vi "Autonomous Independent.vi"() -> ()   [LabVIEW 2014]
doc: "This VI is called when autonomous begins, and will automatically be terminated when autonomous ends. You can carry out timed or sensor driven robot movement independently without needing to return to the caller."
uses:
  <vilib>/Rock Robotics/WPI/Joystick/WPI_JoystickGetSetRefNum.vi
  <vilib>/Rock Robotics/Network Tables/SD Write Numeric Array.vi
  <vilib>/Rock Robotics/Network Tables/SD Read Number.vi
  <vilib>/Rock Robotics/WPI/RobotDrive/WPI_RobotDriveGetSetRefNum.vi
  <vilib>/Rock Robotics/WPI/RobotDrive/WPI_RobotDriveMecanumDrive_Cartesian.vi
panel:
  out "Current Movement, for debugging":T1 {"Z Joystick Value" scale=-1.0..1.0; "Y Joystick Value" scale=1.0..-1.0; "X Joystick Value" scale=-1.0..1.0}
  in  "Array of robot movements":T2(array[cluster]) {"Z Joystick Value" scale=-1.0..1.0; "Y Joystick Value" scale=1.0..-1.0; "X Joystick Value" scale=-1.0..1.0}
  # "Be sure to right-click and choose Data Operations>>Make Current Value default if you want to save the array values with the VI"
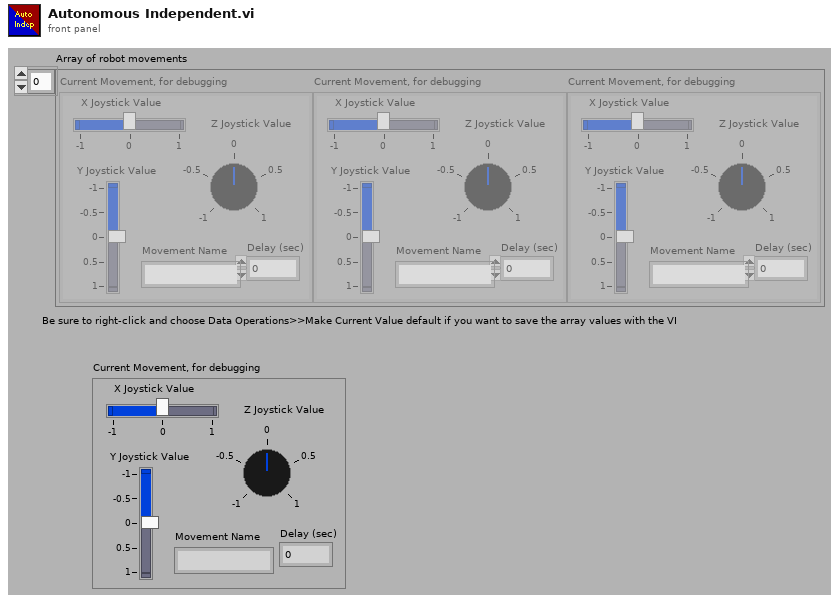
[diagram p1: front panel]
types:
  T1 = cluster{"X Joystick Value":dbl, "Y Joystick Value":dbl, "Z Joystick Value":dbl, "Delay (sec)":dbl, "Movement Name":string}
  T2 = cluster{"X Joystick Value":dbl, "Y Joystick Value":dbl, "Z Joystick Value":dbl, "Delay (sec)":dbl, "Movement Name":string}[]
  T3 = typedef "WPI_JoystickDevRef.ctl" = cluster{"Device":T4}
  T4 = typedef "WPI_JoystickDeviceEnum.ctl" = enum16{"USB 0", "USB 1", "USB 2", "USB 3", "USB 4", "USB 5"}
  T5 = typedef "WPI_RobotDriveDevRef.ctl" = cluster{"DevStatus":errorcluster, "Motors[]":T6[], "Square Inputs":bool, "Max Output":dbl}
  T6 = typedef "WPI_MotorControlDeviceRef.ctl" = cluster{"DeviceStatus":errorcluster, "Type":T7, "PWM":cluster{"Controller":T8, "PWM Channel":T9, "DeadBand":T10}, "CAN":cluster{"Device Number":u8, "Control Mode":T11, "Semaphore":T12, "Max Vout":dbl, "TalonSRX Control Mode":T13}, "Invert":bool, "TransformRef":T14, "InvTransformRef":T14}
  T7 = typedef "WPI_MotorControlType.ctl" = enum16{"PWM", "CAN", "CANTalonSRX"}
  T8 = typedef "FPGA_TypedefDigitalModule.ctl" = enum16{"Controller 1"}
  T9 = typedef "FPGA_DIOPWMChannel.ctl" = enum8{"PWM 0", "PWM 1", "PWM 2", "PWM 3", "PWM 4", "PWM 5", "PWM 6", "PWM 7", "PWM 8", "PWM 9", "PWM MXP 0", "PWM MXP 1", "PWM MXP 2", "PWM MXP 3", "PWM MXP 4", "PWM MXP 5", "PWM MXP 6", "PWM MXP 7", "PWM MXP 8", "PWM MXP 9", "Invalid"}
  T10 = typedef "WPI_PWMDeadband.ctl" = cluster{"Name":string, "maxPositivePwm":i32, "minPositivePwm":i32, "centerPwm":i32, "maxNegativePwm":i32, "minNegativePwm":i32, "angularRange":u16}
  T11 = typedef "WPI_CANJaguar_ControlMode.ctl" = enum8{"Percent VBus", "Current", "Speed", "Position", "Voltage"}
  T12 = typedef "Semaphore RefNum" = refnum<k1>
  T13 = typedef "WPI_CANTalonSRX_APIControlMode.ctl" = enum8{"Percent VBus", "Speed", "Position", "Slave", "Unchanged / Invalid"}
  T14 = typedef "WPI_PWMTransform_ConPane.ctl" = refnum<vi>
  T15 = typedef "WPI_EncoderDevRef.ctl" = cluster{"DevStatus":errorcluster, "EncoderIndex":T16, "CounterIndex":T17, "DistancePerCount":dbl, "Decoding Type":T18}
  T16 = typedef "FPGA_EncoderIdx.ctl" = enum8{"Enc 0", "Enc 1", "Enc 2", "Enc 3", "Enc 4", "Enc 5", "Enc 6", "Enc 7", "Invalid"}
  T17 = typedef "FPGA_CounterCtrSystemIndex.ctl" = enum8{"Ctr 0", "Ctr 1", "Ctr 2", "Ctr 3", "Ctr 4", "Ctr 5", "Ctr 6", "Ctr 7", "Invalid"}
  T18 = typedef "WPI_EncoderType.ctl" = enum16{"1x", "2x", "4x"}
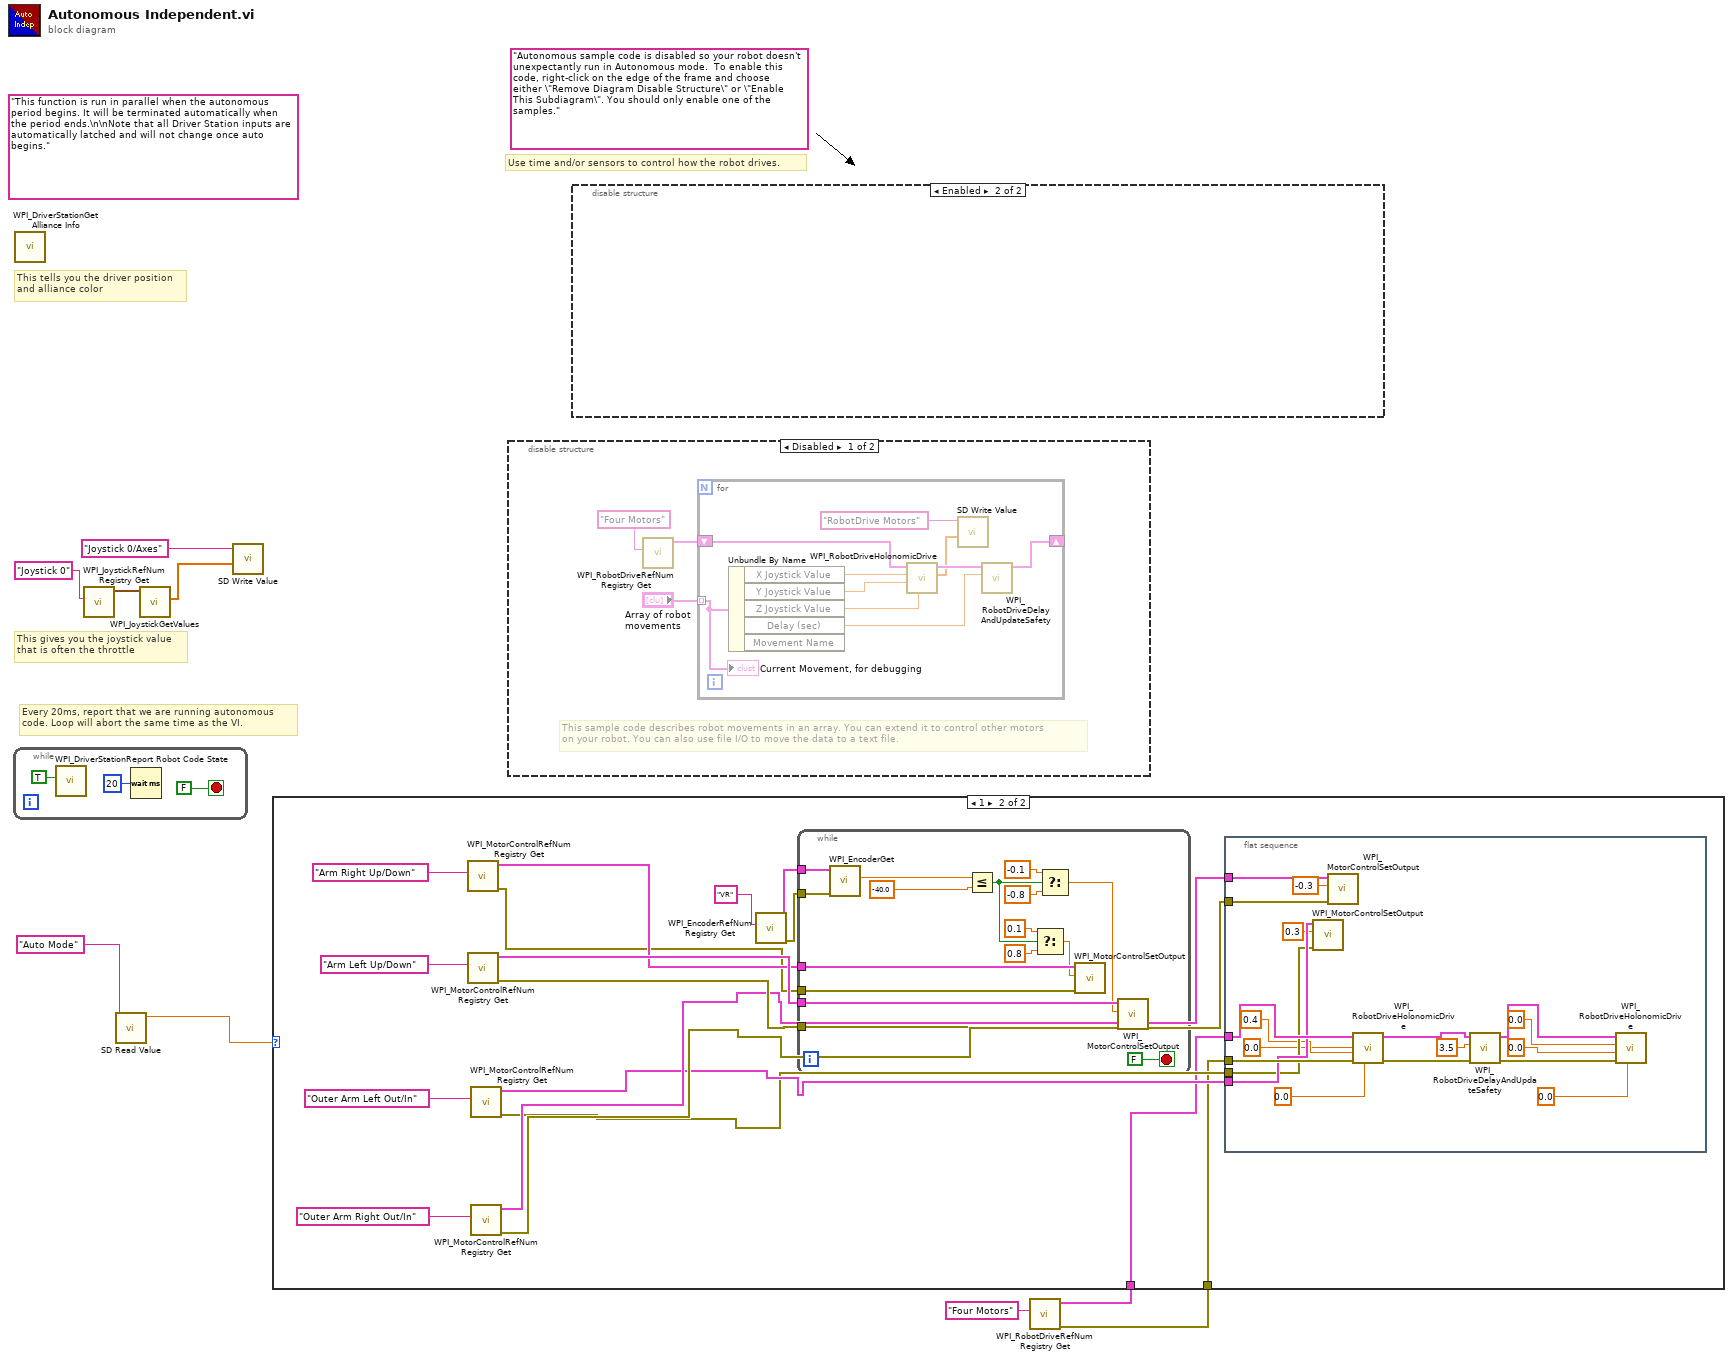
[diagram p0: block diagram]
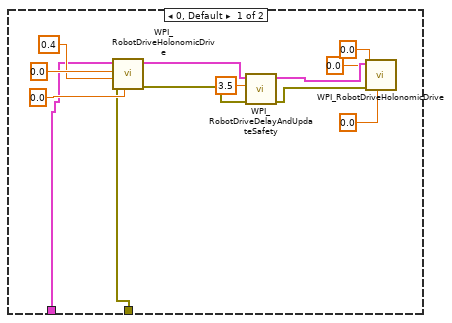
[diagram p2: hidden frame]
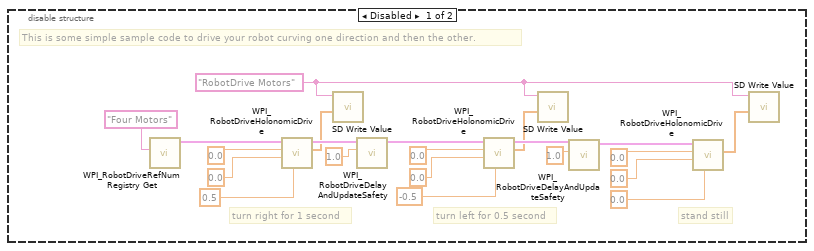
[diagram p4: hidden frame]
diagram:
  (unwired) "Autonomous sample code is disabled so your robot doesn't unexpectantly run in Autonomous mode.  To enable this code, right-click on the edge of the frame and choose either \"Remove Diagram Disable Structure\" or \"Enable This Subdiagram\". You should only enable one of the samples."
  (unwired) "This function is run in parallel when the autonomous period begins. It will be terminated automatically when the period ends.\n\nNote that all Driver Station inputs are automatically latched and will not change once auto begins."
  # "Every 20ms, report that we are running autonomous\ncode. Loop will abort the same time as the VI."
  # "This gives you the joystick value\nthat is often the throttle"
  # "Use time and/or sensors to control how the robot drives."
  # "This tells you the driver position\nand alliance color"
  n1 = while {
    stop <- FALSE stop-if-true
    n2 = call <vilib>:"WPI_DriverStationReport Robot Code State.vi"("Autonomous"=TRUE) -> ()  [unwired: 10 in, 1 out]
    n3 = Wait (ms)(milliseconds to wait=u32 20) -> ()  [unwired: 1 out]
  }
  n4 = call <vilib>:"WPI_DriverStationGet Alliance Info.vi"() -> ()  [unwired: 12 out]
  n5 = call <vilib>:"WPI_JoystickRefNum Registry Get.vi"("refnum name"="Joystick 0") -> ("JoystickDevRef"=w8:T3)  [unwired: 1 in, 9 out]
  n6 = call-poly <vilib>:"SD Read Value.vi"("Name"="Auto Mode") -> ("Numeric"=w5:dbl)  [unwired: 8 in, 2 out]
  n7 = call <vilib>:"WPI_JoystickGetValues.vi"("JoystickDevRef"=w8) -> ("Axes"=w6:dbl[])  [unwired: 6 in, 4 out]
  n8 = call-poly <vilib>:"SD Write Value.vi"("Numeric Array"=w6, "Name"="Joystick 0/Axes") -> ()  [unwired: 8 in, 2 out]
  n9 = disable-structure shown="Disabled" {
    frame Disabled {
      # "This sample code describes robot movements in an array. You can extend it to control other motors\non your robot. You can also use file I/O to move the data to a text file."
      n10 = call <vilib>:"WPI_RobotDriveRefNum Registry Get.vi"("refnum name"="Four Motors") -> ("RobotDriveDevRef"=w14:T5)  [unwired: 1 in, 9 out]
      n11 = for {
        shift-right: [w22] -> _
        shift-left: w14 -> [w23]
        tunnel: "Array of robot movements" -> [w18] mode=indexing
        n12 = Unbundle By Name(w18) -> ("X Joystick Value"=w21:dbl, "Y Joystick Value"=w20:dbl, "Z Joystick Value"=w17:dbl, "Delay (sec)"=w19:dbl)  [unwired: 1 out]
        n13 = call-poly <vilib>:"WPI_RobotDriveHolonomicDrive.vi"("Rotation"=w17, "Y"=w20, "X"=w21, "RobotDriveDevRef"=w23) -> ("Motor Values"=w16:dbl[], "RobotDriveDevRef"=w24:T5)  [unwired: 5 in, 1 out]
        n14 = call-poly <vilib>:"SD Write Value.vi"("Numeric Array"=w16, "Name"="RobotDrive Motors") -> ()  [unwired: 8 in, 2 out]
        n15 = call <vilib>:"WPI_RobotDriveDelayAndUpdateSafety.vi"("Delay (s)"=w19, "RobotDriveDevRef"=w24) -> ("RobotDriveDevRef 2"=w22:T5)  [unwired: 8 in, 1 out]
        "Current Movement, for debugging" <- w18
      }
    }
    frame Enabled {
    }
  }
  n16 = disable-structure shown="Enabled" {
    frame Disabled {
      w32 = "RobotDrive Motors" ("Name")
      # "This is some simple sample code to drive your robot curving one direction and then the other."
      # "stand still"
      # "turn left for 0.5 second"
      # "turn right for 1 second"
      n17 = call <vilib>:"WPI_RobotDriveRefNum Registry Get.vi"("refnum name"="Four Motors") -> ("RobotDriveDevRef"=w33:T5)  [unwired: 1 in, 9 out]
      n18 = call-poly <vilib>:"WPI_RobotDriveHolonomicDrive.vi"("Rotation"=0.5, "Y"=0.0 ("X axis value"), "X"=0.0 ("X axis value"), "RobotDriveDevRef"=w33) -> ("Motor Values"=w28:dbl[], "RobotDriveDevRef"=w40:T5)  [unwired: 5 in, 1 out]
      n19 = call-poly <vilib>:"SD Write Value.vi"("Numeric Array"=w28, "Name"=w32) -> ()  [unwired: 8 in, 2 out]
      n20 = call <vilib>:"WPI_RobotDriveDelayAndUpdateSafety.vi"("Delay (s)"=1.0, "RobotDriveDevRef"=w40) -> ("RobotDriveDevRef 2"=w39:T5)  [unwired: 8 in, 1 out]
      n21 = call-poly <vilib>:"WPI_RobotDriveHolonomicDrive.vi"("Rotation"=-0.5, "Y"=0.0 ("X axis value"), "X"=0.0 ("X axis value"), "RobotDriveDevRef"=w39) -> ("Motor Values"=w27:dbl[], "RobotDriveDevRef"=w38:T5)  [unwired: 5 in, 1 out]
      n22 = call-poly <vilib>:"SD Write Value.vi"("Numeric Array"=w27, "Name"=w32) -> ()  [unwired: 8 in, 2 out]
      n23 = call <vilib>:"WPI_RobotDriveDelayAndUpdateSafety.vi"("Delay (s)"=1.0, "RobotDriveDevRef"=w38) -> ("RobotDriveDevRef 2"=w37:T5)  [unwired: 8 in, 1 out]
      n24 = call-poly <vilib>:"WPI_RobotDriveHolonomicDrive.vi"("Rotation"=0.0 ("X axis value"), "Y"=0.0 ("X axis value"), "X"=0.0 ("X axis value"), "RobotDriveDevRef"=w37) -> ("Motor Values"=w26:dbl[])  [unwired: 5 in, 2 out]
      n25 = call-poly <vilib>:"SD Write Value.vi"("Numeric Array"=w26, "Name"=w32) -> ()  [unwired: 8 in, 2 out]
    }
    frame Enabled {
    }
  }
  n26 = call <vilib>:"WPI_RobotDriveRefNum Registry Get.vi"("refnum name"="Four Motors") -> ("error out"=w2:errorcluster, "RobotDriveDevRef"=w3:T5)  [unwired: 1 in, 8 out]
  n27 = case shown="1" w5 {
    tunnel: w3 -> [w48 w61]
    tunnel: w2 -> [w47 w60]
    frame 0, Default {
      n28 = call-poly <vilib>:"WPI_RobotDriveHolonomicDrive.vi"("Rotation"=0.0, "error in (no error)"=w47, "Y"=0.4 ("Magnitude"), "X"=0.0 ("Direction"), "RobotDriveDevRef"=w48) -> ("error out"=w57:errorcluster, "RobotDriveDevRef"=w56:T5)  [unwired: 4 in, 1 out]
      n29 = call <vilib>:"WPI_RobotDriveDelayAndUpdateSafety.vi"("error in (no error)"=w57, "Delay (s)"=3.5, "RobotDriveDevRef"=w56) -> ("error out"=w59:errorcluster, "RobotDriveDevRef 2"=w58:T5)  [unwired: 7 in]
      n30 = call-poly <vilib>:"WPI_RobotDriveHolonomicDrive.vi"("Rotation"=0.0, "error in (no error)"=w59, "Y"=0.0, "X"=0.0, "RobotDriveDevRef"=w58) -> ()  [unwired: 4 in, 3 out]
    }
    frame 1 {
      n31 = call <vilib>:"WPI_MotorControlRefNum Registry Get.vi"("refnum name"="Arm Right Up/Down") -> ("error out"=w69:errorcluster, "MotorControlDevRef"=w70:T6)  [unwired: 9 in]
      n32 = call <vilib>:"WPI_MotorControlRefNum Registry Get.vi"("refnum name"="Arm Left Up/Down") -> ("error out"=w72:errorcluster, "MotorControlDevRef"=w71:T6)  [unwired: 9 in]
      n33 = call <vilib>:"WPI_MotorControlRefNum Registry Get.vi"("refnum name"="Outer Arm Left Out/In") -> ("error out"=w62:errorcluster, "MotorControlDevRef"=w63:T6)  [unwired: 9 in]
      n34 = call <vilib>:"WPI_MotorControlRefNum Registry Get.vi"("refnum name"="Outer Arm Right Out/In") -> ("error out"=w64:errorcluster, "MotorControlDevRef"=w65:T6)  [unwired: 9 in]
      n35 = call <vilib>:"WPI_EncoderRefNum Registry Get.vi"("refnum name"="VR") -> ("error out"=w67:errorcluster, "EncoderDevRef"=w68:T15)  [unwired: 9 in]
      n36 = while {
        tunnel: w71 -> [w111]
        tunnel: w72 -> [w110]
        tunnel: w70 -> [w109]
        tunnel: w69 -> [w108]
        tunnel: w68 -> [w107]
        tunnel: w67 -> [w106]
        stop <- FALSE stop-if-true
        n37 = call <vilib>:"WPI_EncoderGet.vi"("error in (no error)"=w106, "EncoderDevRef"=w107) -> ("Distance"=w98:dbl)  [unwired: 4 in, 5 out]
        n38 = Less Or Equal?(x=w98, y=-40.0) -> (x <= y?=w104:bool)
        n39 = Select(t=0.1, s=w104, f=0.8 ("Output")) -> (s? t:f=w96:dbl)
        n40 = Select(t=-0.1, s=w104, f=-0.8 ("Output")) -> (s? t:f=w97:dbl)
        n41 = call <vilib>:"WPI_MotorControlSetOutput.vi"("error in (no error)"=w108, "Output"=w96, "MotorControlDevRef"=w109) -> ()  [unwired: 6 in, 3 out]
        n42 = call <vilib>:"WPI_MotorControlSetOutput.vi"("error in (no error)"=w110, "Output"=w97, "MotorControlDevRef"=w111) -> ()  [unwired: 6 in, 3 out]
      }
      n43 = flat-sequence {
        tunnel: w61 -> [w86]
        tunnel: w60 -> [w85]
        tunnel: w65 -> [w84]
        tunnel: w64 -> [w83]
        tunnel: w63 -> [w82]
        tunnel: w62 -> [w81]
        frame #0 {
          n44 = call <vilib>:"WPI_MotorControlSetOutput.vi"("error in (no error)"=w81, "Output"=0.3, "MotorControlDevRef"=w82) -> ()  [unwired: 6 in, 3 out]
          n45 = call <vilib>:"WPI_MotorControlSetOutput.vi"("error in (no error)"=w83, "Output"=-0.3, "MotorControlDevRef"=w84) -> ()  [unwired: 6 in, 3 out]
          n46 = call-poly <vilib>:"WPI_RobotDriveHolonomicDrive.vi"("Rotation"=0.0, "error in (no error)"=w85, "Y"=0.4 ("Magnitude"), "X"=0.0 ("Direction"), "RobotDriveDevRef"=w86) -> ("error out"=w93:errorcluster, "RobotDriveDevRef"=w94:T5)  [unwired: 4 in, 1 out]
          n47 = call <vilib>:"WPI_RobotDriveDelayAndUpdateSafety.vi"("error in (no error)"=w93, "Delay (s)"=3.5, "RobotDriveDevRef"=w94) -> ("error out"=w90:errorcluster, "RobotDriveDevRef 2"=w91:T5)  [unwired: 7 in]
          n48 = call-poly <vilib>:"WPI_RobotDriveHolonomicDrive.vi"("Rotation"=0.0, "error in (no error)"=w90, "Y"=0.0 ("Direction"), "X"=0.0 ("Magnitude"), "RobotDriveDevRef"=w91) -> ()  [unwired: 4 in, 3 out]
        }
      }
    }
  }
